vi "Disconnect.vi"(8 "error in (no error)":errorcluster, 11 "MSOX6004 in":refnum<class "MSOX6004.lvclass">) -> (0 "error out":errorcluster, 3 "MSOX6004 out":refnum<class "MSOX6004.lvclass">)   [LabVIEW 2018, in "MSOX6004.lvlib" / "MSOX6004.lvclass"]
doc: "This Override method is used finalize the communication session with the Oscope instrument."
uses:
  MSOX6004.lvclass
  MSOX6004.lvclass/MSOX6004.ctl
  <instrlib>/Keysight InfiniiVision/Keysight InfiniiVision.lvlib
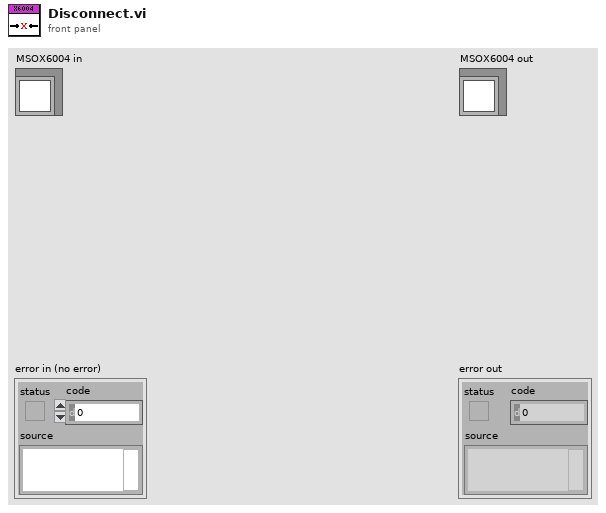
[diagram p1: front panel]
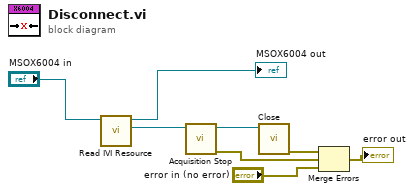
[diagram p0: block diagram]
diagram:
  n1 = call "Read IVI Resource.vi"("MSOX6004 in"="MSOX6004 in") -> ("IVI Resource"=w4:refnum<k15>, "MSOX6004 out"=→"MSOX6004 out":refnum<class "MSOX6004.lvclass">)  [unwired: 8 in, 1 out]
  n2 = call <instrlib>:"Acquisition Stop.vi"("instrument handle"=w4) -> ("error out"=w2:errorcluster, "instrument handle out"=w3:refnum<k15>)  [unwired: 9 in]
  n3 = call <instrlib>:"Close.vi"("instrument handle"=w3) -> ("error out"=w6:errorcluster)  [unwired: 10 in]
  n4 = Merge Errors(w6, w2, "error in (no error)") -> (→"error out":errorcluster)
